vi "4145 Take Measurement.vi"(8 "error in":T2, 9 "wait for SRQ?":bool, 10 "measurement command (single:0)":u16(ring) items=["SINGLE", "REPEAT", "APPEND", "STOP"], 11 "4145_GPIB_COM_in":T1={"Address_string"="17", "timeout ms"=25000, "Terminator"=",", "LoggerQueue"=refnum}) -> (0 "error out":T2, 3 "4145_GPIB_COM_out":T1={"Address_string"="17", "timeout ms"=25000, "Terminator"=",", "LoggerQueue"=refnum})   [LabVIEW 2014]
doc: "This VI can send the four measurment control commands to the instrument. These commands control the starting and stopping of the measurements. The four choices are:\n0: single\n1: repeat\n2: append\n3: stop\n\nThis VI also gives you the chance to set Data Ready Service Request ON if you wish an interrupt to be sent when measurement data is valid. The output buffer is cleared before this occurs if this option is chosen. DRI is set back to off after the measurement is done."
uses:
  typedef/4145_GPIB_Com.ctl
  typedef/4145_que_msg.ctl
  typedef/4145 command enum.ctl
panel:
  out "concatenated string":string
  # "yes\n\nno"
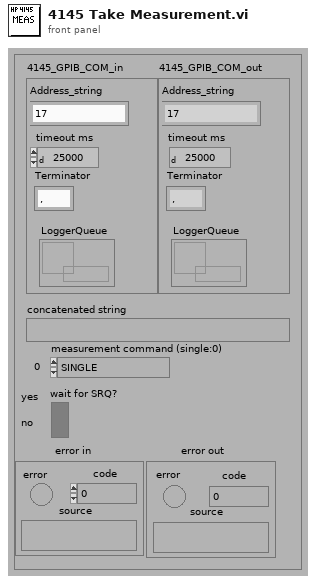
[diagram p1: front panel]
types:
  T1 = typedef "4145_GPIB_Com.ctl" = cluster{"Address_string":string, "timeout ms":u32, "Terminator":string, "LoggerQueue":refnum<queue>}
  T2 = cluster{"error":bool, "code":i32, "source":string}
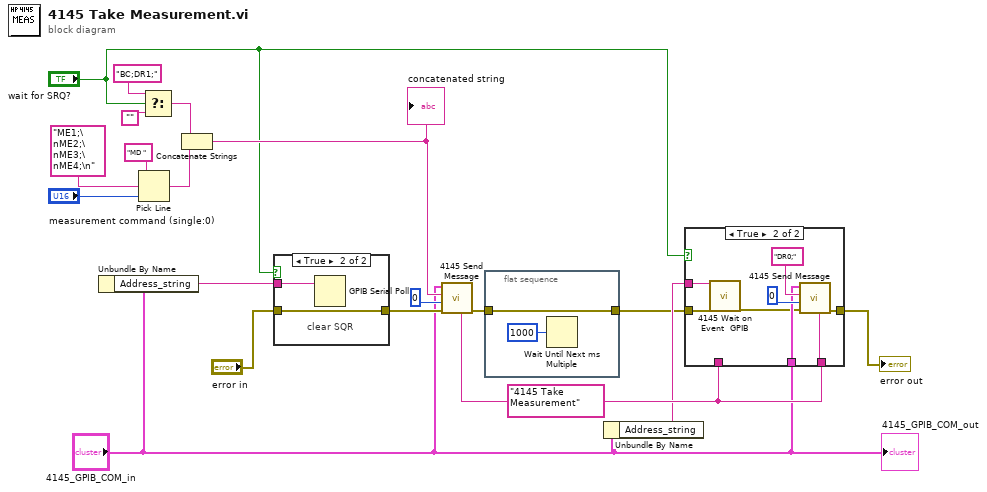
[diagram p0: block diagram]
diagram:
  w4 = "4145 Take Measurement"
  n1 = Unbundle By Name("4145_GPIB_COM_in") -> ("Address_string"=w6:string)
  n2 = Pick Line(string ("")="MD ", multi-line string="ME1;\nME2;\nME3;\nME4;\n", line index="measurement command (single:0)") -> (output string=w12:string)
  n3 = Select(t="BC;DR1;", s="wait for SRQ?", f="") -> (s? t:f=w11:string)
  n4 = Concatenate Strings(w11, w12) -> (w15:string)
  "concatenated string" <- w15
  n5 = case shown="True" "wait for SRQ?" {
    tunnel: w6 -> [_ w22]
    tunnel: "error in" -> [w20 w21]
    tunnel: [w20 w21] -> w8
    frame False {
    }
    frame True {
      # "clear SQR"
      n6 = GPIB Serial Poll(0:w22) -> ()  [unwired: 1 in, 3 out]
    }
  }
  n7 = call "4145 Send Message.vi"("source IN"=w4, "error in"=w8, "write mode (set END:0)"=0, "write buffer IN"=w15, "4145_GPIB_COM_IN"="4145_GPIB_COM_in") -> ("error out"=w5:T2)  [unwired: 3 in, 3 out]
  n8 = flat-sequence {
    tunnel: w5 -> [w23]
    tunnel: [w23] -> w1
    frame #0 {
      n9 = Wait Until Next ms Multiple(millisecond multiple=u32 1000) -> ()  [unwired: 1 out]
    }
  }
  n10 = Unbundle By Name("4145_GPIB_COM_in") -> ("Address_string"=w2:string)
  n11 = case shown="True" "wait for SRQ?" {
    tunnel: [w25 w29] -> w10
    tunnel: w4 -> [_ w30]
    tunnel: "4145_GPIB_COM_in" -> [_ w31]
    tunnel: w4 -> [_ _]
    tunnel: w2 -> [_ w28]
    tunnel: w1 -> [w25 w27]
    frame False {
    }
    frame True {
      n12 = call "4145 Wait on Event  GPIB .vi"("Address"=w28, "error in"=w27) -> ("error out"=w26:errorcluster)  [unwired: 15 in, 2 out]
      n13 = call "4145 Send Message.vi"("source IN"=w30, "error in"=w26, "write mode (set END:0)"=0, "write buffer IN"="DR0;", "4145_GPIB_COM_IN"=w31) -> ("error out"=w29:T2)  [unwired: 3 in, 3 out]
    }
  }
  "error out" <- w10
  "4145_GPIB_COM_out" <- "4145_GPIB_COM_in"
